vi "A170316-11_Auto.vi"() -> ()   [LabVIEW 2020]
uses:
  Global_Variable/A170316-11.vi
  Global_Variable/Global.vi
  Database/Global1.vi
  <vilib>/addons/database/Connection.llb/DB Tools Open Connec (String).vi
  <vilib>/addons/database/NI_Database_API.lvlib
panel:
  in  "前序OK？_ECU":string
  in  "前序OK？":string
  out "磨合次数":i32
  in  "判定结果":bool[][](array[boolean])=[[TRUE]]
  in  "STEP3":string
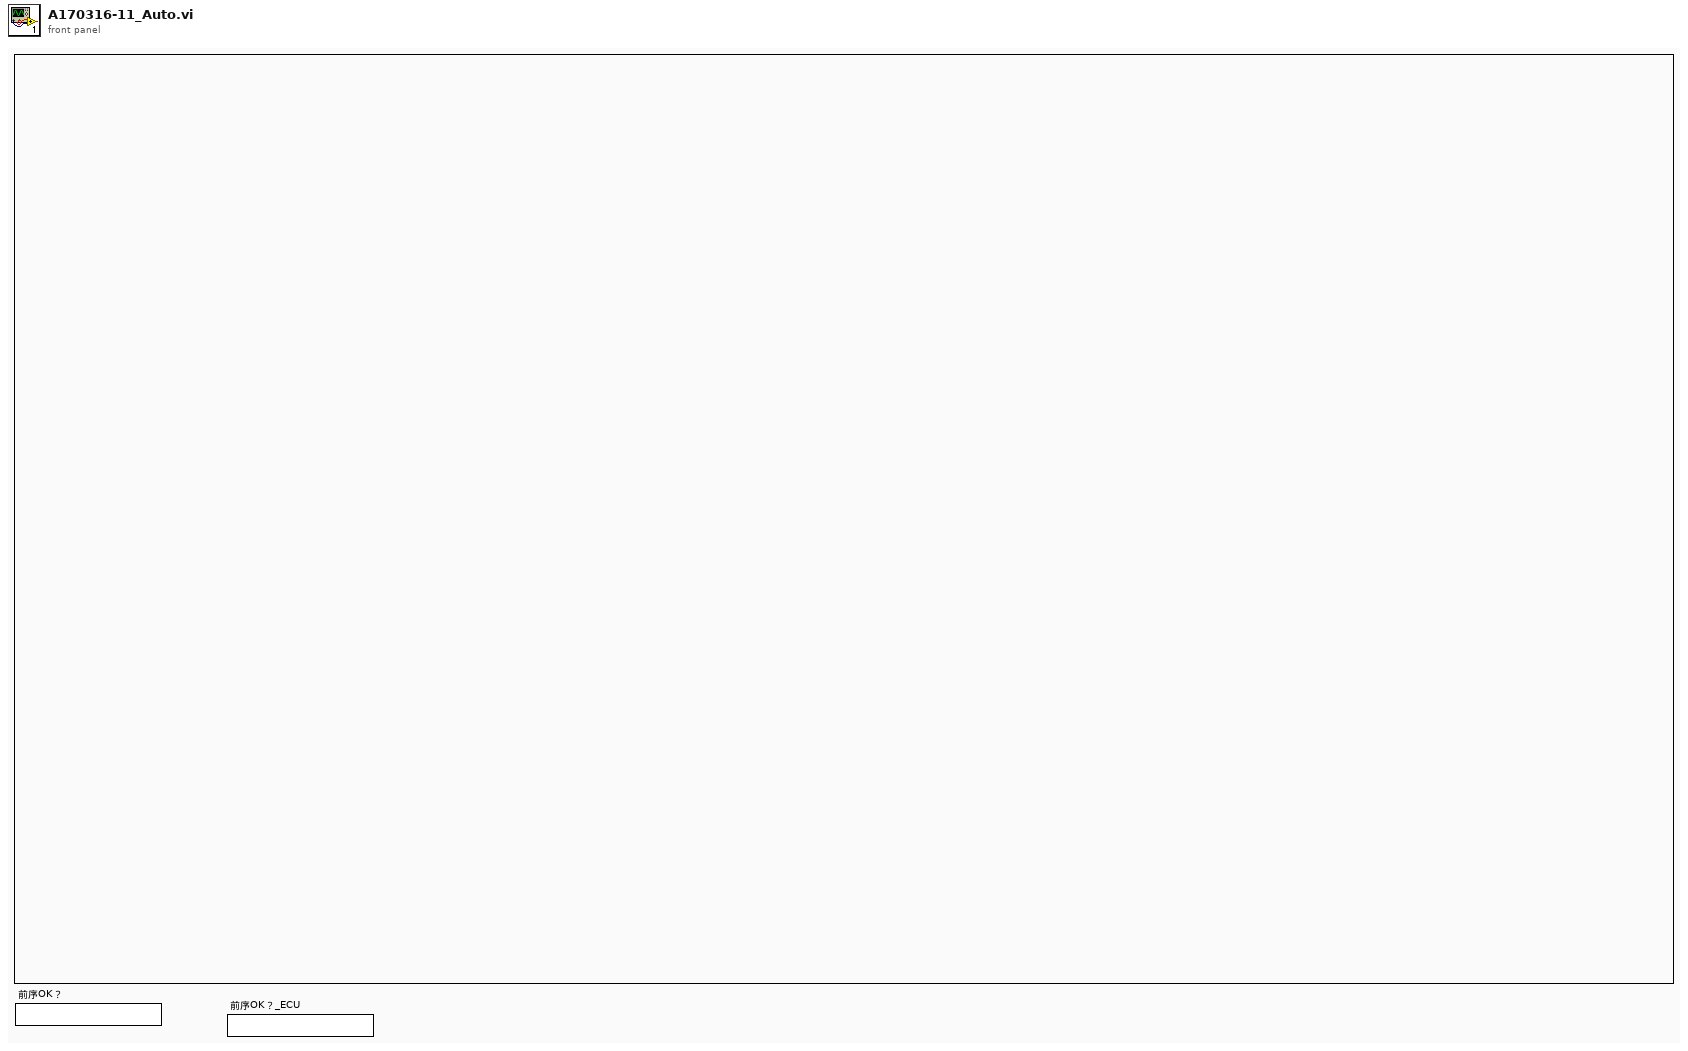
[diagram p1: front panel]
types:
  T1 = cluster{i64, i64, i64, "生产结果":string, "result string":string}
  T2 = cluster{i64, i64, i64, "生产结果":string, "result string":string}[]
  T3 = typedef "NI_Database_API.lvlib/Conn ObjectReference.ctl" = refnum<k1>
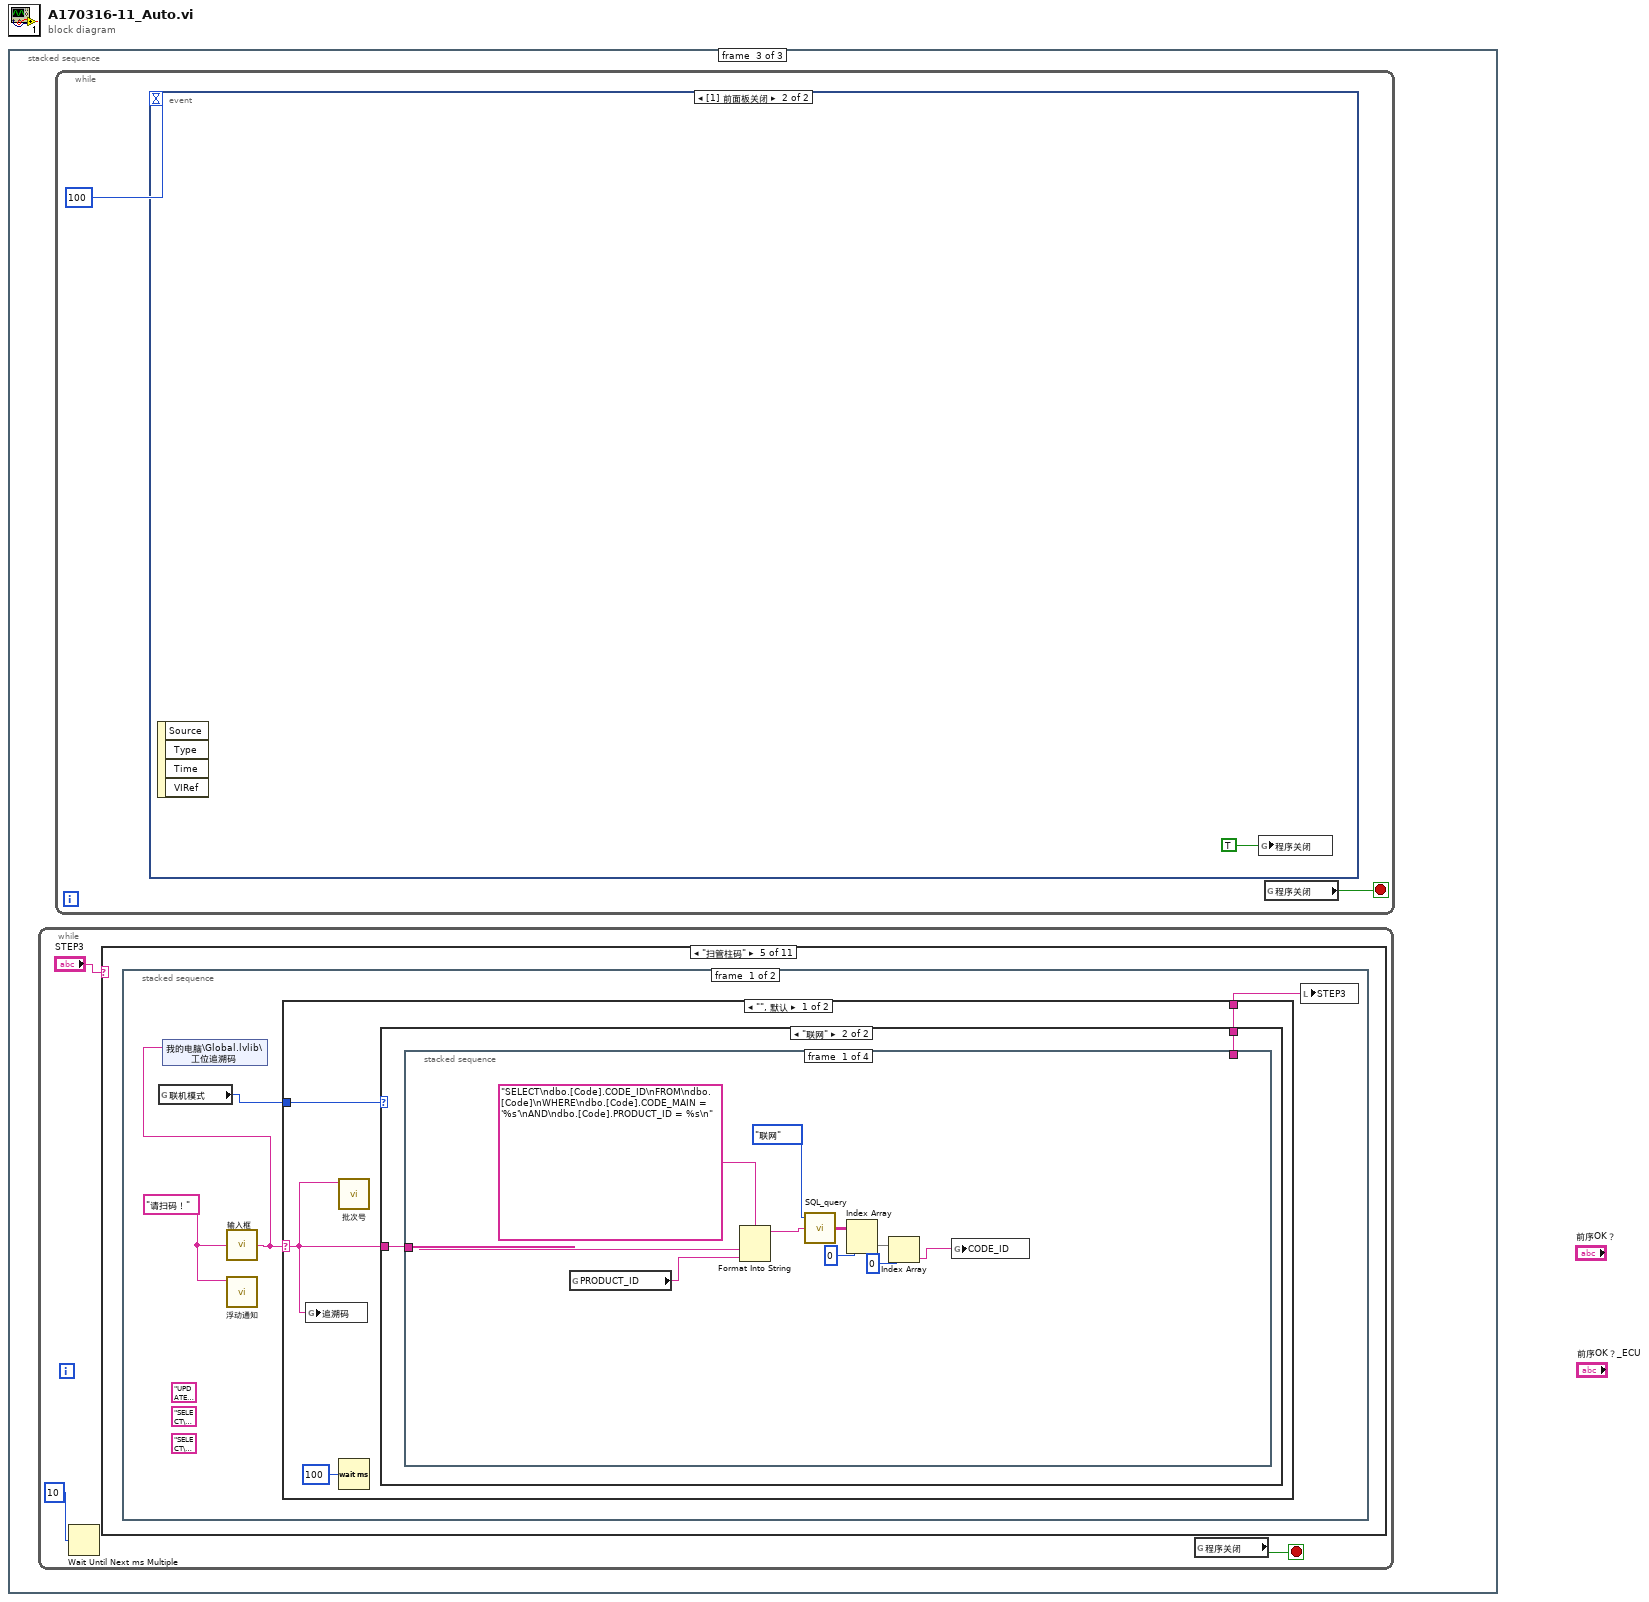
[diagram p0: block diagram]
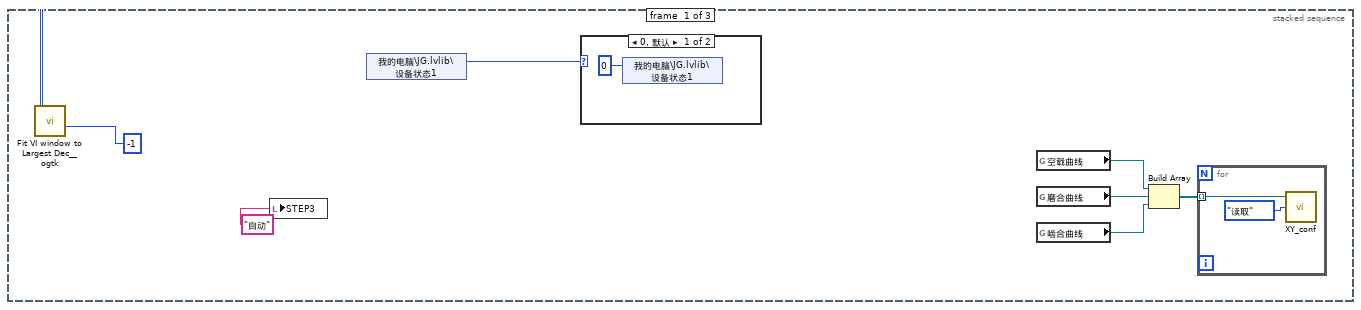
[diagram p2: hidden frame]
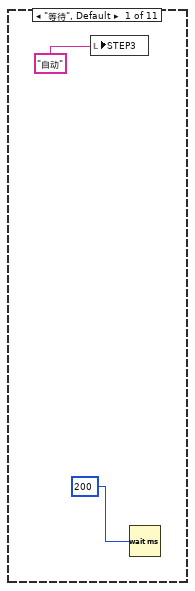
[diagram p5: hidden frame]
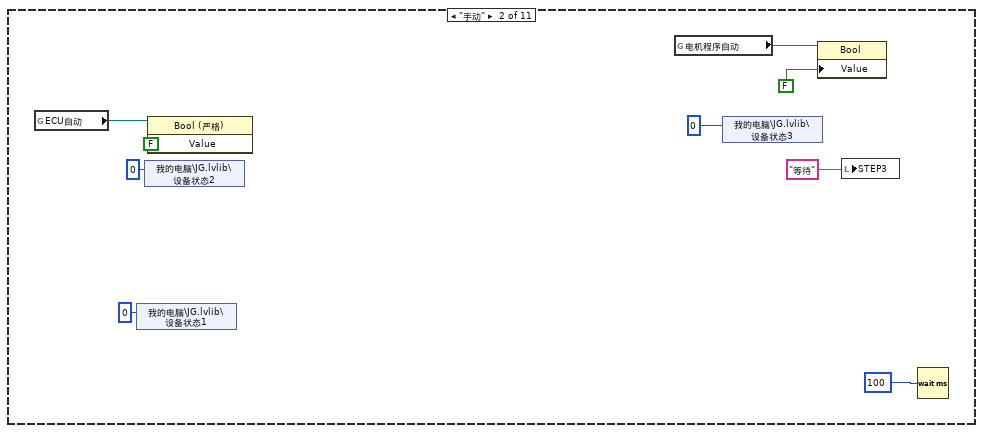
[diagram p6: hidden frame]
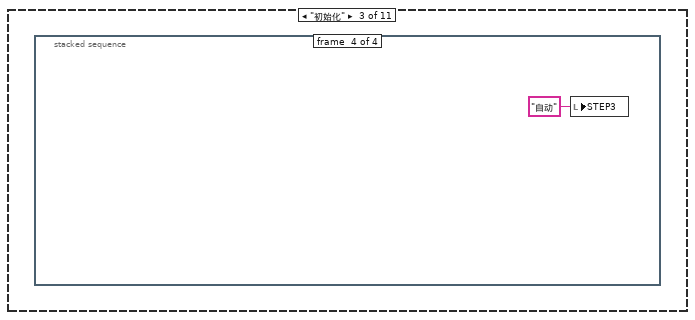
[diagram p7: hidden frame]
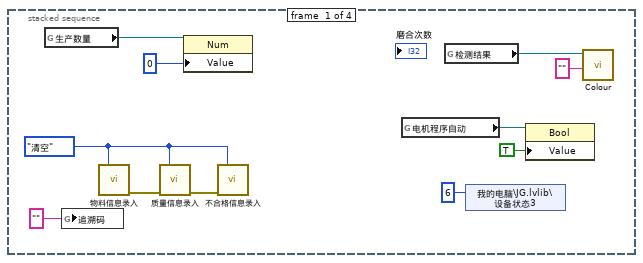
[diagram p8: hidden frame]
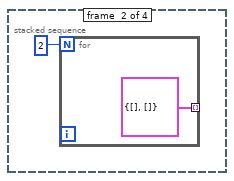
[diagram p9: hidden frame]
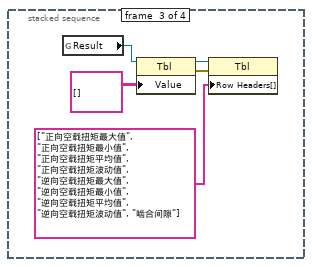
[diagram p10: hidden frame]
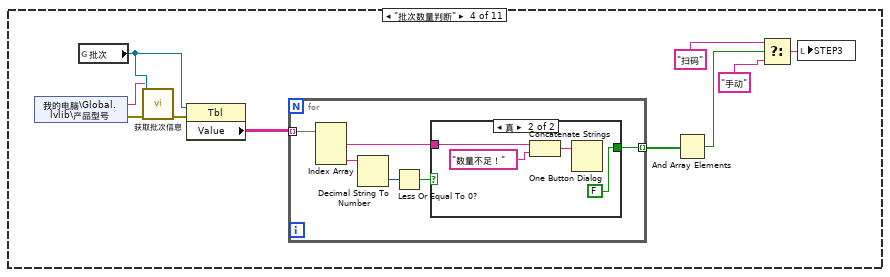
[diagram p11: hidden frame]
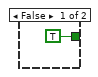
[diagram p12: hidden frame]
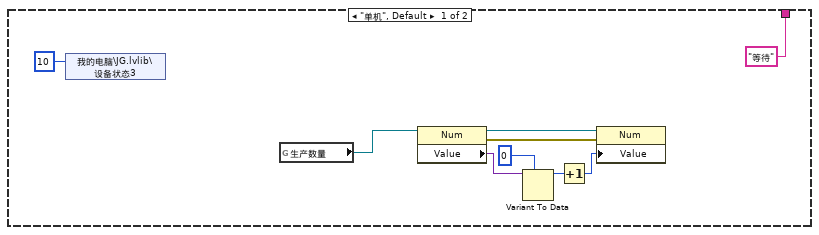
[diagram p13: hidden frame]
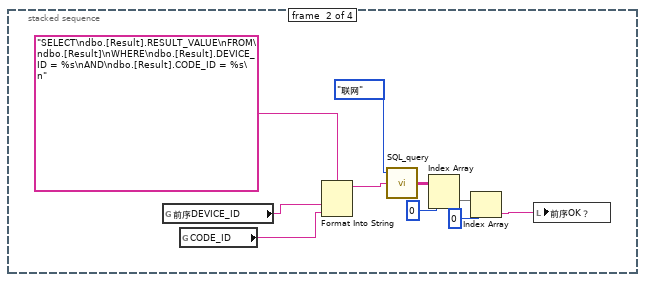
[diagram p14: hidden frame]
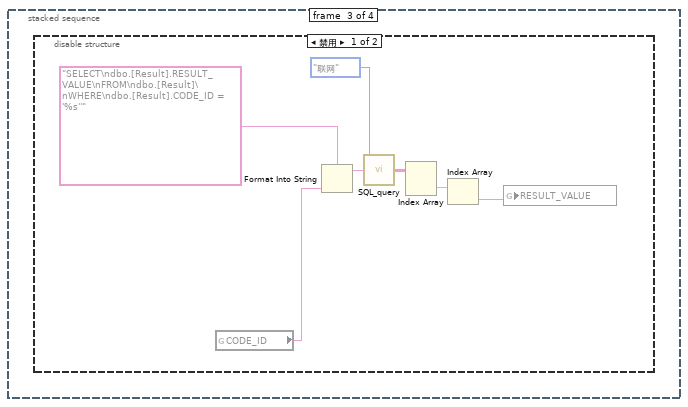
[diagram p15: hidden frame]
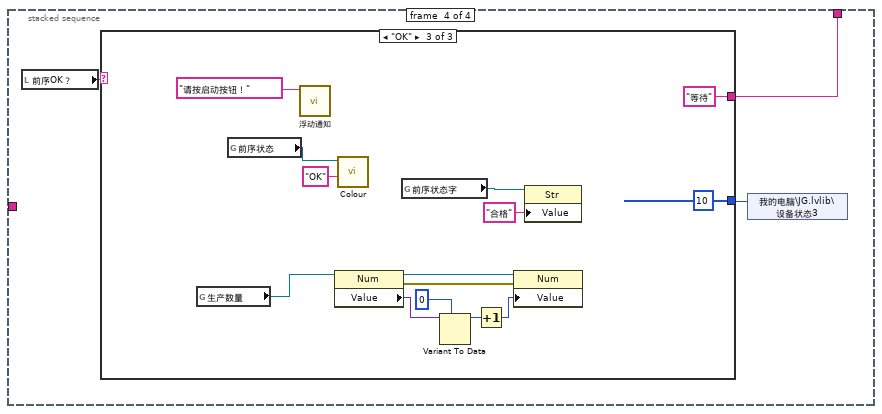
[diagram p17: hidden frame]
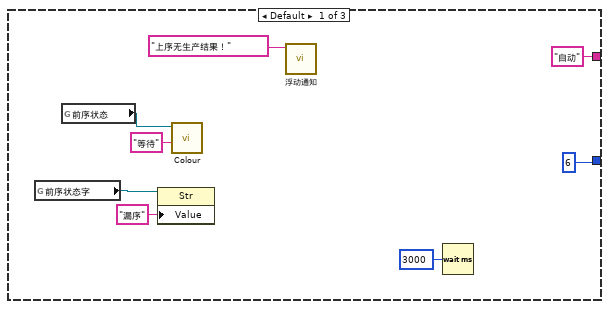
[diagram p18: hidden frame]
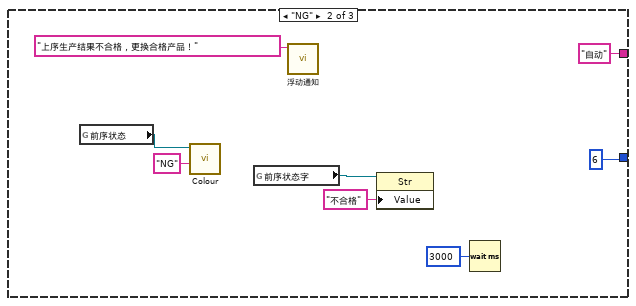
[diagram p19: hidden frame]
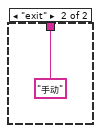
[diagram p20: hidden frame]
diagram:
  n1 = stacked-sequence {
    frame #0 {
      n2 = call <userlib>:"Fit VI window to Largest Dec__ogtk.vi"("border spacing (2 px)"=-1) -> ()  [unwired: 5 in, 2 out]
      n3 = local write "STEP3"("自动" ("STEP")) -> ()
      n4 = shared-variable "我的电脑\\JG.lvlib\\设备状态1"() -> (w5:i16)  [unwired: 1 in, 1 out]
      n5 = case shown="0, 默认" w5 {
        frame 0, Default {
          n6 = shared-variable "我的电脑\\JG.lvlib\\设备状态1"(i16 0 ("设备状态")) -> ()  [unwired: 1 in, 1 out]
        }
        frame 3721..3723 {
        }
      }
      n7 = global read "A170316-11.vi" "空载曲线"() -> (w1:refnum<vi>)
      n8 = global read "A170316-11.vi" "磨合曲线"() -> (w2:refnum<vi>)
      n9 = global read "A170316-11.vi" "啮合曲线"() -> (w3:refnum<vi>)
      n10 = Build Array(w1, w2, w3) -> (w6:refnum<vi>[])
      n11 = for {
        tunnel: w6 -> [w10] mode=indexing
        n12 = call "XY_conf.vi"("方式"=enum16{"写入", "读取"}."读取", "XY图引用"=w10) -> ()  [unwired: 3 in, 1 out]
      }
    }
    frame #1 {
    }
    frame #2 {
      n13 = while {
        stop <- w12 stop-if-true
        n14 = Wait Until Next ms Multiple(millisecond multiple=u32 10 ("毫秒倍数")) -> ()  [unwired: 1 out]
        n15 = case shown="\"扫管柱码\"" "STEP3" {
          frame "等待", Default {
            n16 = local write "STEP3"("自动" ("STEP")) -> ()
            n17 = Wait (ms)(milliseconds to wait=u32 200 ("等待时间（毫秒）")) -> ()  [unwired: 1 out]
          }
          frame "手动" {
            n18 = global read "Global.vi" "ECU自动"() -> (w19:refnum<vi>)
            n19 = shared-variable "我的电脑\\JG.lvlib\\设备状态1"(u16 0 ("设备状态")) -> ()  [unwired: 1 in, 1 out]
            n20 = shared-variable "我的电脑\\JG.lvlib\\设备状态2"(u16 0 ("设备状态")) -> ()  [unwired: 1 in, 1 out]
            n21 = property class="Bool (严格)"(reference=w19, "Value"=FALSE) -> ()  [unwired: 1 in, 2 out]
            n22 = global read "Global.vi" "电机程序自动"() -> (w22:refnum<vi>)
            n23 = shared-variable "我的电脑\\JG.lvlib\\设备状态3"(u16 0 ("设备状态")) -> ()  [unwired: 1 in, 1 out]
            n24 = property class="Bool"(reference=w22, "Value"=FALSE) -> ()  [unwired: 1 in, 2 out]
            n25 = local write "STEP3"("等待" ("STEP")) -> ()
            n26 = Wait (ms)(milliseconds to wait=u32 100 ("等待时间（毫秒）")) -> ()  [unwired: 1 out]
          }
          frame "初始化" {
            n27 = stacked-sequence {
              frame #0 {
                w34 = enum16{"录入", "清空"}."清空" ("功能")
                n28 = global read "Global.vi" "生产数量"() -> (w28:refnum<vi>)
                n29 = global write "Global1.vi" "追溯码"("" ("传感器码")) -> ()
                n30 = call "物料信息录入.vi"("功能"=w34) -> ("错误输出"=w33:errorcluster)  [unwired: 14 in]
                n31 = call "质量信息录入.vi"("功能"=w34, "错误输入（无错误）"=w33) -> ("错误输出"=w35:errorcluster)  [unwired: 13 in]
                n32 = property class="Num"(reference=w28, "Value"=0 ("磨合次数")) -> ()  [unwired: 1 in, 2 out]
                n33 = call "不合格信息录入.vi"("功能"=w34, "错误输入（无错误）"=w35) -> ()  [unwired: 13 in, 1 out]
                n34 = global read "Global.vi" "电机程序自动"() -> (w32:refnum<vi>)
                n35 = global read "Global.vi" "检测结果"() -> (w30:refnum<vi>)
                n36 = shared-variable "我的电脑\\JG.lvlib\\设备状态3"(i16 6 ("设备状态")) -> ()  [unwired: 1 in, 1 out]
                n37 = property class="Bool"(reference=w32, "Value"=TRUE) -> ()  [unwired: 1 in, 2 out]
                n38 = call "Colour.vi"("result"="", "colourRef"=w30) -> ()  [unwired: 9 in, 1 out]
              }
              frame #1 {
                n39 = for {
                  N: 2 -> [_]
                  tunnel: [cluster{dbl[], dbl[]} {[], []}] -> _ mode=indexing
                }
              }
              frame #2 {
                n40 = global read "Global.vi" "Result"() -> (w40:refnum<vi>)
                n41 = property class="Tbl"(reference=w40, "Value"=string[][] []) -> (reference out=w41:refnum<vi>, error out=w42:errorcluster)  [unwired: 1 in]
                n42 = property class="Tbl"(reference=w41, error in=w42, "Row Headers[]"=string[] ["正向空载扭矩最大值", "正向空载扭矩最小值", "正向空载扭矩平均值", "正向空载扭矩波动值", "逆向空载扭矩最大值", "逆向空载扭矩最小值", "逆向空载扭矩平均值", "逆向空载扭矩波动值", "啮合间隙"] ("列首字符串[]")) -> ()  [unwired: 2 out]
              }
              frame #3 {
                n43 = local write "STEP3"("自动" ("STEP")) -> ()
              }
            }
          }
          frame "批次数量判断" {
            n44 = shared-variable "我的电脑\\Global.lvlib\\产品型号"() -> (w49:string, error out=w52:errorcluster)  [unwired: 1 in]
            n45 = global read "Global.vi" "批次"() -> (w50:refnum<vi>)
            n46 = call "获取批次信息.vi"("error in (no error)"=w52, "产品型号"=w49, "Tbl引用句柄"=w50) -> ("error out"=w51:errorcluster)  [unwired: 7 in, 1 out]
            n47 = property class="Tbl"(reference=w50, error in=w51) -> ("Value"=w53:string[][])  [unwired: 2 out]
            n48 = for {
              tunnel: w53 -> [w59] mode=indexing
              tunnel: [w54] -> w48 mode=indexing
              n49 = Index Array(array=w59) -> (element #1=w55:string, element #3=w58:string)  [unwired: 3 in, 1 out]
              n50 = Decimal String To Number(string=w58) -> (number=w57:i32)  [unwired: 2 in, 1 out]
              n51 = Less Or Equal To 0?(x=w57) -> (x <= 0?=w56:bool)
              n52 = case shown="真" w56 {
                tunnel: w55 -> [_ w64]
                tunnel: [TRUE FALSE] -> w54
                frame False {
                }
                frame True {
                  n53 = Concatenate Strings(w64, "数量不足！" ("字符串")) -> (w62:string)
                  n54 = One Button Dialog(message=w62) -> ()  [unwired: 1 in, 1 out]
                }
              }
            }
            n55 = And Array Elements(Boolean array=w48) -> (logical AND=w47:bool)
            n56 = Select(t="扫码" ("STEP"), s=w47, f="手动" ("STEP")) -> (s? t:f=w44:string)
            n57 = local write "STEP3"(w44) -> ()
          }
          frame "扫管柱码" {
            n58 = stacked-sequence {
              frame #0 {
                (unwired) "SELECT\ndbo.[Code].CODE_ID,\ndbo.[Code].CODE_MAIN,\ndbo.[Code].PRODUCT_ID\n\nFROM\ndbo.[Code].CODE_MAIN = 'MACAU3001'" ("格式字符串")
                (unwired) "SELECT\n*\nFROM\ndbo.[Code]\nWHERE\ndbo.[Code].CODE_MAIN = 'MACAU3001'" ("格式字符串")
                (unwired) "UPDATE\ndbo.[Code]\nSET dbo.[Code].CODE_SENSOR = 'henglong'\nWHERE\ndbo.[Code].CODE_MAIN = 'MACAU3001'\n" ("格式字符串")
                w68 = "请扫码！" ("提示信息")
                n59 = global read "Global1.vi" "联机模式"() -> (w66:enum16{"单机", "联网"})
                n60 = call "输入框.vi"("提示信息"=w68) -> ("条形码输出"=w65:string)
                n61 = shared-variable "我的电脑\\Global.lvlib\\工位追溯码"(w65) -> ()  [unwired: 1 in, 1 out]
                n62 = call "浮动通知.vi"("通知内容"=w68) -> ()  [unwired: 11 in]
                n63 = case shown="\"\", 默认" w65 {
                  selector: w65 -> [w69 _]
                  tunnel: [w71 "手动"] -> w67
                  tunnel: w66 -> [w70 _]
                  frame "", Default {
                    n64 = global write "Global1.vi" "追溯码"(w69) -> ()
                    n65 = call "批次号.vi"("批次码"=w69) -> ()  [unwired: 11 in]
                    n66 = Wait (ms)(milliseconds to wait=u32 100 ("等待时间（毫秒）")) -> ()  [unwired: 1 out]
                    n67 = case shown="\"联网\"" w70 {
                      tunnel: w69 -> [_ w83]
                      tunnel: ["等待" ("State(s) in Front (\"\")") w82] -> w71
                      frame "单机", Default {
                        n68 = shared-variable "我的电脑\\JG.lvlib\\设备状态3"(i16 10 ("设备状态控制字")) -> ()  [unwired: 1 in, 1 out]
                        n69 = global read "Global.vi" "生产数量"() -> (w75:refnum<vi>)
                        n70 = property class="Num"(reference=w75) -> (reference out=w73:refnum<vi>, error out=w77:errorcluster, "Value"=w78:variant)  [unwired: 1 in]
                        n71 = Variant To Data(type=u32 0, Variant=w78) -> (data=w79:u32)  [unwired: 1 in, 1 out]
                        n72 = Increment(x=w79) -> (x+1=w80:u32)
                        n73 = property class="Num"(reference=w73, error in=w77, "Value"=w80) -> ()  [unwired: 2 out]
                      }
                      frame "联网" {
                        n74 = stacked-sequence {
                          tunnel: w83 -> [w90 _ _ _]
                          tunnel: [_ _ _ w112] -> w82
                          frame #0 {
                            n75 = global read "Global1.vi" "PRODUCT_ID"() -> (w87:string)
                            n76 = Format Into String(format string="SELECT\ndbo.[Code].CODE_ID\nFROM\ndbo.[Code]\nWHERE\ndbo.[Code].CODE_MAIN = '%s'\nAND\ndbo.[Code].PRODUCT_ID = %s\n" ("格式字符串"), w90, w87) -> (resulting string=w89:string)  [unwired: 2 in, 1 out]
                            n77 = call "SQL_query.vi"("SQL query"=w89, "联机模式"=enum16{"单机", "联网"}."联网") -> ("data"=w93:string[][])  [unwired: 1 in, 2 out]
                            n78 = Index Array(array=w93, index (row)=0 ("索引 (行)")) -> (element=w92:string[])  [unwired: 1 in]
                            n79 = Index Array(array=w92, index=0 ("索引")) -> (element=w84:string)
                            n80 = global write "Global1.vi" "CODE_ID"(w84) -> ()
                          }
                          frame #1 {
                            n81 = global read "Global1.vi" "前序DEVICE_ID"() -> (w95:string)
                            n82 = global read "Global1.vi" "CODE_ID"() -> (w94:string)
                            n83 = Format Into String(format string="SELECT\ndbo.[Result].RESULT_VALUE\nFROM\ndbo.[Result]\nWHERE\ndbo.[Result].DEVICE_ID = %s\nAND\ndbo.[Result].CODE_ID = %s\n" ("格式字符串"), w95, w94) -> (resulting string=w100:string)  [unwired: 2 in, 1 out]
                            n84 = call "SQL_query.vi"("SQL query"=w100, "联机模式"=enum16{"单机", "联网"}."联网") -> ("data"=w103:string[][])  [unwired: 1 in, 2 out]
                            n85 = Index Array(array=w103, index (row)=0 ("索引 (行)")) -> (element=w102:string[])  [unwired: 1 in]
                            n86 = Index Array(array=w102, index=0 ("索引")) -> (element=w96:string)
                            n87 = local write "前序OK？"(w96) -> ()
                          }
                          frame #2 {
                            n88 = disable-structure shown="禁用" {
                              frame Disabled {
                                n89 = global read "Global1.vi" "CODE_ID"() -> (w105:string)
                                n90 = Format Into String(format string="SELECT\ndbo.[Result].RESULT_VALUE\nFROM\ndbo.[Result]\nWHERE\ndbo.[Result].CODE_ID = '%s''" ("格式字符串"), w105) -> (resulting string=w107:string)  [unwired: 2 in, 1 out]
                                n91 = call "SQL_query.vi"("SQL query"=w107, "联机模式"=enum16{"单机", "联网"}."联网") -> ("data"=w110:string[][])  [unwired: 1 in, 2 out]
                                n92 = Index Array(array=w110) -> (element=w108:string[])  [unwired: 2 in]
                                n93 = Index Array(array=w108) -> (element=w109:string)  [unwired: 1 in]
                                n94 = global write "Global1.vi" "RESULT_VALUE"(w109) -> ()
                              }
                              frame Enabled {
                              }
                            }
                          }
                          frame #3 {
                            n95 = local read "前序OK？"() -> (w111:string)
                            n96 = case shown="\"OK\"" w111 {
                              tunnel: [i16 6 ("设备状态控制字") i16 6 ("设备状态控制字") i16 10 ("设备状态控制字")] -> w113
                              tunnel: ["自动" "自动" "等待"] -> w112
                              frame Default {
                                n97 = global read "Global1.vi" "前序状态字"() -> (w115:refnum<vi>)
                                n98 = global read "Global1.vi" "前序状态"() -> (w117:refnum<vi>)
                                n99 = property class="Str"(reference=w115, "Value"="漏序" ("值")) -> ()  [unwired: 1 in, 2 out]
                                n100 = call "Colour.vi"("result"="等待", "colourRef"=w117) -> ()  [unwired: 9 in, 1 out]
                                n101 = call "浮动通知.vi"("通知内容"="上序无生产结果！" ("Status")) -> ()  [unwired: 11 in]
                                n102 = Wait (ms)(milliseconds to wait=u32 3000) -> ()  [unwired: 1 out]
                              }
                              frame "NG" {
                                n103 = global read "Global1.vi" "前序状态"() -> (w125:refnum<vi>)
                                n104 = call "Colour.vi"("result"="NG", "colourRef"=w125) -> ()  [unwired: 9 in, 1 out]
                                n105 = global read "Global1.vi" "前序状态字"() -> (w123:refnum<vi>)
                                n106 = call "浮动通知.vi"("通知内容"="上序生产结果不合格，更换合格产品！" ("Status")) -> ()  [unwired: 11 in]
                                n107 = property class="Str"(reference=w123, "Value"="不合格" ("值")) -> ()  [unwired: 1 in, 2 out]
                                n108 = Wait (ms)(milliseconds to wait=u32 3000) -> ()  [unwired: 1 out]
                              }
                              frame "OK" {
                                n109 = global read "Global.vi" "生产数量"() -> (w141:refnum<vi>)
                                n110 = global read "Global1.vi" "前序状态"() -> (w133:refnum<vi>)
                                n111 = call "浮动通知.vi"("通知内容"="请按启动按钮！" ("Status")) -> ()  [unwired: 11 in]
                                n112 = property class="Num"(reference=w141) -> (reference out=w142:refnum<vi>, error out=w140:errorcluster, "Value"=w139:variant)  [unwired: 1 in]
                                n113 = call "Colour.vi"("result"="OK", "colourRef"=w133) -> ()  [unwired: 9 in, 1 out]
                                n114 = global read "Global1.vi" "前序状态字"() -> (w131:refnum<vi>)
                                n115 = Variant To Data(type=u32 0, Variant=w139) -> (data=w138:u32)  [unwired: 1 in, 1 out]
                                n116 = Increment(x=w138) -> (x+1=w137:u32)
                                n117 = property class="Num"(reference=w142, error in=w140, "Value"=w137) -> ()  [unwired: 2 out]
                                n118 = property class="Str"(reference=w131, "Value"="合格" ("值")) -> ()  [unwired: 1 in, 2 out]
                              }
                            }
                            n119 = shared-variable "我的电脑\\JG.lvlib\\设备状态3"(w113) -> ()  [unwired: 1 in, 1 out]
                          }
                        }
                      }
                    }
                  }
                  frame "exit" {
                  }
                }
                n120 = local write "STEP3"(w67) -> ()
              }
              frame #1 {
                n121 = Wait (ms)(milliseconds to wait=u32 100 ("等待时间（毫秒）")) -> ()  [unwired: 1 out]
              }
            }
          }
          frame "扫电机码" {
            n122 = stacked-sequence {
              frame #0 {
                w146 = "请扫管柱码！" ("提示信息")
                n123 = call "输入框.vi"("提示信息"=w146) -> ("条形码输出"=w147:string)
                n124 = call "浮动通知.vi"("通知内容"=w146) -> ()  [unwired: 11 in]
                n125 = case shown="\"\", 默认" w147 {
                  selector: w147 -> [w149 _]
                  tunnel: [w150 "手动"] -> w148
                  frame "", Default {
                    n126 = global read "Global1.vi" "联机模式"() -> (w151:enum16{"单机", "联网"})
                    n127 = shared-variable "我的电脑\\Global.lvlib\\电机码"(w149) -> ()  [unwired: 1 in, 1 out]
                    n128 = case shown="\"联网\"" w151 {
                      tunnel: w149 -> [_ _]
                      tunnel: ["等待" ("State(s) in Front (\"\")") w155] -> w150
                      frame "单机", Default {
                        n129 = shared-variable "我的电脑\\JG.lvlib\\设备状态3"(i16 35 ("设备状态控制字")) -> ()  [unwired: 1 in, 1 out]
                        n130 = Wait (ms)(milliseconds to wait=u32 100 ("等待时间（毫秒）")) -> ()  [unwired: 1 out]
                      }
                      frame "联网" {
                        n131 = stacked-sequence {
                          tunnel: [_ _ "等待" ("State(s) in Front (\"\")")] -> w155
                          frame #0 {
                          }
                          frame #1 {
                          }
                          frame #2 {
                            n132 = shared-variable "我的电脑\\JG.lvlib\\设备状态3"(i16 35 ("设备状态控制字")) -> ()  [unwired: 1 in, 1 out]
                          }
                        }
                      }
                    }
                  }
                  frame "exit" {
                  }
                }
                n133 = local write "STEP3"(w148) -> ()
              }
              frame #1 {
                n134 = Wait (ms)(milliseconds to wait=u32 100 ("等待时间（毫秒）")) -> ()  [unwired: 1 out]
              }
            }
          }
          frame "录入批次" {
            n135 = shared-variable "我的电脑\\Global.lvlib\\产品型号"() -> (w161:string)  [unwired: 1 in, 1 out]
            n136 = call "更新批次.vi"("型号"=w161) -> ("error out"=w162:errorcluster)  [unwired: 10 in]
            n137 = call "更新易损件.vi"("error in (no error)"=w162) -> ("error out"=w165:errorcluster)  [unwired: 10 in]
            n138 = global read "Global.vi" "批次"() -> (w163:refnum<vi>)
            n139 = property class="Tbl"(reference=w163, error in=w165) -> ("Value"=w164:string[][])  [unwired: 2 out]
            n140 = for {
              tunnel: w164 -> [w168] mode=indexing
              n141 = Index Array(array=w168) -> (element #1=w167:string, element #2=w166:string)  [unwired: 2 in]
              n142 = call "物料信息录入.vi"("物料名称"=w167, "功能"=enum16{"录入", "清空"}."录入", "物料编码"=w166) -> ()  [unwired: 12 in, 1 out]
            }
            n143 = local write "STEP3"("等待" ("STEP")) -> ()
          }
          frame "自动" {
            n144 = shared-variable "我的电脑\\JG.lvlib\\设备状态3"() -> (w170:i16)  [unwired: 1 in, 1 out]
            n145 = case shown="100, 200" w170 {
              frame Default {
              }
              frame -128 {
                n146 = call "浮动通知.vi"("通知内容"="复位中……" ("Status")) -> ()  [unwired: 11 in]
                n147 = global read "Global.vi" "电机程序自动"() -> (w172:refnum<vi>)
                n148 = property class="Bool"(reference=w172, "Value"=FALSE) -> ()  [unwired: 1 in, 2 out]
              }
              frame 5 {
                n149 = call "浮动通知.vi"("通知内容"="复位完成" ("Status")) -> ()  [unwired: 11 in]
              }
              frame 6 {
                n150 = local write "STEP3"("扫管柱码") -> ()
              }
              frame 0 {
              }
              frame 7 {
                n151 = global read "Global.vi" "电机结果显示"() -> (w179:refnum<vi>)
                n152 = shared-variable "我的电脑\\Global.lvlib\\工位追溯码"("" ("传感器码")) -> ()  [unwired: 1 in, 1 out]
                n153 = property class="Str"(reference=w179, "Value"="..." ("结果显示")) -> (reference out=w178:refnum<vi>)  [unwired: 1 in, 1 out]
                n154 = property class="Str"(reference=w178, "Text.TextColor"=u32 16776960) -> ()  [unwired: 1 in, 2 out]
                n155 = local write "STEP3"("扫管柱码" ("STEP3")) -> ()
              }
              frame 8 {
                n156 = call "浮动通知.vi"("通知内容"="程序停止！" ("Status")) -> ()  [unwired: 11 in]
              }
              frame 9 {
                n157 = call "浮动通知.vi"("通知内容"="套花键中" ("Status")) -> ()  [unwired: 11 in]
              }
              frame 11 {
                n158 = call "浮动通知.vi"("通知内容"="主码更新到打标机！" ("Status")) -> ()  [unwired: 11 in]
              }
              frame 12 {
                n159 = call "浮动通知.vi"("通知内容"="已更新到打标机！" ("Status")) -> ()  [unwired: 11 in]
              }
              frame 100, 200 {
                n160 = global read "Global.vi" "电机结果显示"() -> (w189:refnum<vi>)
                n161 = property class="Str"(reference=w189, "Value"=" ..." ("结果显示")) -> (reference out=w188:refnum<vi>)  [unwired: 1 in, 1 out]
                n162 = property class="Str"(reference=w188, "Text.TextColor"=u32 9567230) -> ()  [unwired: 1 in, 2 out]
                n163 = call "浮动通知.vi"("通知内容"="移栽进！" ("Status")) -> ()  [unwired: 11 in]
              }
              frame 300 {
                n164 = call "浮动通知.vi"("通知内容"="防护门下降！" ("Status")) -> ()  [unwired: 11 in]
              }
              frame 400 {
                n165 = call "浮动通知.vi"("通知内容"="启动达标！" ("Status")) -> ()  [unwired: 11 in]
              }
              frame 401 {
                n166 = call "浮动通知.vi"("通知内容"="激光打标中！" ("Status")) -> ()  [unwired: 11 in]
              }
              frame 500 {
                n167 = call "浮动通知.vi"("通知内容"="打标完成！" ("Status")) -> ()  [unwired: 11 in]
              }
              frame 600 {
                n168 = call "浮动通知.vi"("通知内容"="返回！" ("Status")) -> ()  [unwired: 11 in]
              }
              frame 601 {
                n169 = global read "Global1.vi" "联机模式"() -> (w196:enum16{"单机", "联网"})
                n170 = Wait (ms)(milliseconds to wait=u32 500 ("等待时间（毫秒）")) -> ()  [unwired: 1 out]
                n171 = case shown="\"单机\", 默认" w196 {
                  frame "单机", Default {
                    n172 = global read "Global.vi" "检测结果"() -> (w205:refnum<vi>)
                    n173 = call "浮动通知.vi"("通知内容"="产品合格！" ("Status")) -> ()  [unwired: 11 in]
                    n174 = call "Colour.vi"("result"="OK", "colourRef"=w205) -> ()  [unwired: 9 in, 1 out]
                    n175 = global read "Global.vi" "电机结果显示"() -> (w202:refnum<vi>)
                    n176 = property class="Str"(reference=w202, "Value"="OK" ("结果显示")) -> (reference out=w201:refnum<vi>)  [unwired: 1 in, 1 out]
                    n177 = shared-variable "我的电脑\\JG.lvlib\\设备状态3"(i16 6 ("设备状态")) -> ()  [unwired: 1 in, 1 out]
                    n178 = property class="Str"(reference=w201, "Text.TextColor"=u32 65344) -> ()  [unwired: 1 in, 2 out]
                  }
                  frame "联网" {
                    n179 = global read "Global.vi" "检测结果"() -> (w214:refnum<vi>)
                    n180 = global write "Global1.vi" "生产结果"("OK" ("电机工位生产结果")) -> ()
                    n181 = call "浮动通知.vi"("通知内容"="产品合格！" ("Status")) -> ()  [unwired: 11 in]
                    n182 = call "Colour.vi"("result"="OK", "colourRef"=w214) -> ()  [unwired: 9 in, 1 out]
                    n183 = global read "Global.vi" "电机结果显示"() -> (w212:refnum<vi>)
                    n184 = property class="Str"(reference=w212, "Value"="OK" ("结果显示")) -> (reference out=w209:refnum<vi>)  [unwired: 1 in, 1 out]
                    n185 = property class="Str"(reference=w209, "Text.TextColor"=u32 6618880) -> ()  [unwired: 1 in, 2 out]
                    n186 = local write "STEP3"("录入数据库" ("STEP3")) -> ()
                  }
                }
              }
              frame 201 {
                n187 = global read "Global.vi" "检测结果"() -> (w220:refnum<vi>)
                n188 = call "Colour.vi"("result"="NG", "colourRef"=w220) -> ()  [unwired: 9 in, 1 out]
                n189 = call "浮动通知.vi"("通知内容"="产品不合格！" ("Status")) -> ()  [unwired: 11 in]
                n190 = global read "Global.vi" "电机结果显示"() -> (w219:refnum<vi>)
                n191 = property class="Str"(reference=w219, "Value"="NG" ("结果显示")) -> (reference out=w218:refnum<vi>)  [unwired: 1 in, 1 out]
                n192 = property class="Str"(reference=w218, "Text.TextColor"=u32 16711680) -> ()  [unwired: 1 in, 2 out]
              }
              frame 999 {
                n193 = call "浮动通知.vi"("通知内容"="请重新安装固定螺栓！" ("Status")) -> ()  [unwired: 11 in]
                n194 = shared-variable "我的电脑\\JG.lvlib\\设备状态3"(i16 40 ("设备状态")) -> ()  [unwired: 1 in, 1 out]
              }
              frame 1024 {
                n195 = call "浮动通知.vi"("通知内容"="急停！" ("Status")) -> ()  [unwired: 11 in]
                n196 = global read "Global.vi" "电机程序自动"() -> (w225:refnum<vi>)
                n197 = property class="Bool"(reference=w225, "Value"=FALSE) -> ()  [unwired: 1 in, 2 out]
              }
              frame 3721 {
                n198 = local write "STEP3"("不合格锁定" ("STEP")) -> ()
                n199 = call "浮动通知.vi"("通知内容"="产品不合格程序锁定！" ("Status")) -> ()  [unwired: 11 in]
              }
              frame 3722 {
                n200 = global read "Global.vi" "电机程序自动"() -> (w230:refnum<vi>)
                n201 = call "浮动通知.vi"("通知内容"="授权成功，请复位！" ("Status")) -> ()  [unwired: 11 in]
                n202 = property class="Bool"(reference=w230, "Value"=FALSE) -> ()  [unwired: 1 in, 2 out]
              }
              frame 3723 {
                n203 = call "浮动通知.vi"("通知内容"="请取出不合格产品并摆放至不合格品区！" ("Status")) -> ()  [unwired: 11 in]
              }
            }
          }
          frame "录入数据库" {
            n204 = stacked-sequence {
              frame #0 {
                n205 = Get Date/Time String(date format (0)=enum16{"short", "long", "abbreviated"}."short" ("日期格式(0)"), want seconds? (F)=FALSE ("需要秒？(F)")) -> (date string=w242:string, time string=w243:string)  [unwired: 1 in]
                n206 = global read "Global1.vi" "DEVICE_ID"() -> (w246:string)
                n207 = global read "Global1.vi" "USER_ID"() -> (w244:string)
                n208 = global read "Global1.vi" "CODE_ID"() -> (w245:string)
                n209 = global read "Global1.vi" "生产结果"() -> (w237:string)
                n210 = Concatenate Strings(w242, " " ("字符串"), w243) -> (w238:string)
                n211 = Decimal String To Number(string=w246, default (0L)=i64 0 ("默认(0 I32)")) -> (number=w235:i64)  [unwired: 1 in, 1 out]
                n212 = Decimal String To Number(string=w244, default (0L)=i64 0 ("默认(0 I32)")) -> (number=w234:i64)  [unwired: 1 in, 1 out]
                n213 = Decimal String To Number(string=w245, default (0L)=i64 0 ("默认(0 I32)")) -> (number=w233:i64)  [unwired: 1 in, 1 out]
                n214 = global read "Global1.vi" "联机模式"() -> (w253:enum16{"单机", "联网"})
                n215 = Search and Replace String(replace all?=TRUE ("替换全部？(F)"), input string=w238, search string="/" ("替换字符串(\"\")"), replace string="-" ("替换字符串(\"\")")) -> (result string=w236:string)  [unwired: 4 in, 3 out]
                n216 = Bundle(w235, w234, w233, "生产结果"=w237, "result string"=w236) -> (w259:T1)  [unwired: 1 in]
                n217 = call "GetSQLstring.vi"("联机模式"=w253) -> ("错误输出"=w256:errorcluster, "连接字符串"=w255:string)  [unwired: 9 in]
                n218 = Build Array(w259) -> (w260:T2)
                n219 = call-poly <vilib>:"DB Tools Open Connection.vi"("error in (no error)"=w256, "connection information"=w255) -> ("error out"=w254:errorcluster, "connection reference"=w257:T3)  [unwired: 6 in]
                n220 = for {
                  tunnel: w260 -> [w265] mode=indexing
                  tunnel: w257 -> [w263]
                  shift-right: [w261] -> w258
                  shift-left: w254 -> [w268]
                  w264 = string[] ["DEVICE_ID", "USER_ID", "CODE_ID", "RESULT_VALUE", "RESULT_TIME"] ("columns")
                  w266 = "Result" ("table")
                  n221 = call <vilib>:"DB Tools Insert Data.vi"("data"=w265, "error in (no error)"=w268, "columns"=w264, "table"=w266, "connection reference"=w263) -> ("error out"=w267:errorcluster, "connection reference out"=w262:T3)  [unwired: 5 in]
                  n222 = case shown="错误" w267 {
                    selector: w267 -> [w269 w290]
                    tunnel: w264 -> [_ w287]
                    tunnel: w262 -> [w270 w279]
                    tunnel: w266 -> [_ w291]
                    tunnel: w265 -> [_ w283]
                    tunnel: [w270 w278] -> _
                    tunnel: [w269 w277] -> w261
                    frame No Error {
                    }
                    frame Error {
                      n223 = Array Subset(array=w287, index=3 ("长度"), length=2 ("长度")) -> (w288:string[])
                      n224 = Unbundle(w283) -> (w272:i64, w275:i64, "生产结果"=w282:string, "result string"=w281:string)  [unwired: 1 out]
                      n225 = Number To Decimal String(number=w275) -> (decimal integer string=w276:string)  [unwired: 1 in]
                      n226 = Number To Decimal String(number=w272) -> (decimal integer string=w271:string)  [unwired: 1 in]
                      n227 = Concatenate Strings("WHERE CODE_ID =" ("condition"), w276, "AND DEVICE_ID = ", w271) -> (w284:string)
                      n228 = Bundle("生产结果"=w282, "result string"=w281) -> (w280:cluster{"生产结果":string, "result string":string})  [unwired: 1 in]
                      n229 = call <vilib>:"Clear Errors.vi"("error in (no error)"=w290) -> ("error out"=w289:errorcluster)  [unwired: 5 in, 1 out]
                      n230 = call <vilib>:"DB Tools Update Data.vi"("condition"=w284, "data"=w280, "error in (no error)"=w289, "columns"=w288, "table"=w291, "connection reference"=w279) -> ("error out"=w277:errorcluster, "connection reference out"=w278:T3)  [unwired: 4 in]
                    }
                  }
                }
                n231 = call <vilib>:"Simple Error Handler.vi"("error in (no error)"=w258) -> ()  [unwired: 4 in, 5 out]
              }
              frame #1 {
              }
              frame #2 {
              }
              frame #3 {
                n232 = call "浮动通知.vi"("通知内容"="数据录入成功！" ("Status")) -> ()  [unwired: 11 in]
                n233 = shared-variable "我的电脑\\JG.lvlib\\设备状态3"(i16 6 ("设备状态")) -> ()  [unwired: 1 in, 1 out]
                n234 = local write "STEP3"("自动" ("STEP")) -> ()
                n235 = Wait (ms)(milliseconds to wait=u32 1000 ("等待时间（毫秒）")) -> ()  [unwired: 1 out]
              }
            }
          }
          frame "不合格锁定" {
            n236 = call "临时授权.vi"() -> ("授权成功"=w297:bool)  [unwired: 11 in]
            n237 = case shown="真" w297 {
              frame False {
              }
              frame True {
                n238 = local write "STEP3"("报表" ("STEP")) -> ()
                n239 = shared-variable "我的电脑\\JG.lvlib\\设备状态1"(i16 3722 ("设备状态")) -> ()  [unwired: 1 in, 1 out]
              }
            }
            n240 = Wait (ms)(milliseconds to wait=u32 100 ("等待时间（毫秒）")) -> ()  [unwired: 1 out]
          }
          frame "报表" {
            n241 = call "浮动通知.vi"("通知内容"="报表生成中" ("Status")) -> ()  [unwired: 11 in]
            n242 = shared-variable "我的电脑\\Global.lvlib\\工位追溯码"() -> (w309:string)  [unwired: 1 in, 1 out]
            n243 = Index Array(array="判定结果", index (col)=1 ("禁用的索引 (列)")) -> (element=w304:bool[])  [unwired: 1 in]
            n244 = And Array Elements(Boolean array=w304) -> (logical AND=w301:bool)
            n245 = shared-variable "我的电脑\\Global.lvlib\\联机模式"() -> (w306:i16)  [unwired: 1 in, 1 out]
            n246 = case shown="真" w301 {
              frame False {
              }
              frame True {
                n247 = global read "Global.vi" "生产数量"() -> (w318:refnum<vi>)
                n248 = property class="Num"(reference=w318) -> (reference out=w317:refnum<vi>, error out=w316:errorcluster, "Value"=w315:variant)  [unwired: 1 in]
                n249 = Variant To Data(type=u32 0, Variant=w315) -> (data=w314:u32)  [unwired: 1 in, 1 out]
                n250 = Increment(x=w314) -> (x+1=w313:u32)
                n251 = property class="Num"(reference=w317, error in=w316, "Value"=w313) -> ()  [unwired: 2 out]
              }
            }
            n252 = call "Report_A170316-11.vi"("文件重命名"=TRUE, "文件名称"=w309, "布尔数组"="判定结果") -> ("error out"=w307:errorcluster)  [unwired: 8 in]
            n253 = case shown="0, 默认" w306 {
              tunnel: w307 -> [_ w319]
              frame 0, Default {
              }
              frame 1 {
                n254 = call "上传数据库.vi"("错误输入"=w319) -> ()  [unwired: 10 in, 1 out]
              }
            }
            n255 = shared-variable "我的电脑\\JG.lvlib\\设备状态1"() -> (w300:i16)  [unwired: 1 in, 1 out]
            n256 = case shown="3721..3723" w300 {
              frame Default {
                n257 = local write "STEP3"("初始化" ("STEP")) -> ()
              }
              frame 3721..3723 {
                n258 = local write "STEP3"("等待" ("STEP")) -> ()
              }
            }
          }
        }
        n259 = global read "Global.vi" "程序关闭"() -> (w12:bool)
      }
      n260 = while {
        stop <- w320 stop-if-true
        n261 = event shown="[1] 前面板关闭" {
          selector: _ -> [_ _]
          dyn-events: _ -> [_ _]
          timeout: 100 -> [_ _]
          event Timeout {
            n262 = event-data() -> ()  [unwired: 1 in, 3 out]
            n263 = stacked-sequence {
              frame #0 {
                n264 = shared-variable "我的电脑\\JG.lvlib\\错误代码"() -> (w322:u16)  [unwired: 1 in, 1 out]
                n265 = feedback #1() -> (w332:u16)  [unwired: 1 in]
                n266 = feedback-in #1(w322) -> ()
                n267 = Greater Or Equal?(x=w322, y=i16 5000) -> (x >= y?=w330:bool)
                n268 = Less?(x=w322, y=i16 5200) -> (x < y?=w331:bool)
                n269 = Equal?(x=w322, y=w332) -> (x = y?=w329:bool)
                n270 = global read "Global.vi" "报警图标"() -> (w324:refnum<vi>)
                n271 = And(x=w330, y=w331) -> (x .and. y?=w323:bool)
                n272 = property class="Bool"(reference=w324, "Value"=w323) -> ()  [unwired: 1 in, 2 out]
                n273 = Bundle By Name(cluster=errorcluster {"status"=FALSE, "code"=0, "source"=""} ("错误常量"), "status"=w323, "code"=w322) -> (w328:errorcluster)
                n274 = case shown="真" w329 {
                  tunnel: w328 -> [w337 _]
                  frame False {
                    n275 = call "报警处理.vi"("错误常量"=w337) -> ()  [unwired: 9 in, 2 out]
                  }
                  frame True {
                  }
                }
                n276 = case shown="0" w322 {
                  frame 0 {
                    n277 = global read "Global.vi" "报警图标"() -> (w333:refnum<vi>)
                    n278 = property class="Bool"(reference=w333, "Visible"=FALSE ("可见")) -> ()  [unwired: 1 in, 2 out]
                  }
                  frame 1, Default {
                    n279 = global read "Global.vi" "报警图标"() -> (w336:refnum<vi>)
                    n280 = property class="Bool"(reference=w336, "Visible"=TRUE ("可见")) -> ()  [unwired: 1 in, 2 out]
                  }
                }
              }
              frame #1 {
                n281 = disable-structure shown="启用" {
                  frame Disabled {
                    n282 = global read "Global.vi" "ECU自动"() -> (w338:refnum<vi>)
                    n283 = property class="Bool (严格)"(reference=w338) -> ("Value"=w339:bool)  [unwired: 1 in, 2 out]
                    n284 = Variant To Data(type=FALSE, Variant=w339) -> (data=w341:bool)  [unwired: 1 in, 1 out]
                    n285 = case shown="真" w341 {
                      selector: w341 -> [w343 _]
                      frame False {
                        n286 = call <userlib>:"Boolean Trigger__ogtk.vi"("Boolean Input"=w343) -> ("Rising Edge"=w342:bool)  [unwired: 1 in, 1 out]
                        n287 = case shown="假" w342 {
                          frame False {
                          }
                          frame True {
                            n288 = local write "STEP3"("手动" ("STEP")) -> ()
                          }
                        }
                      }
                      frame True {
                        n289 = shared-variable "我的电脑\\JG.lvlib\\设备状态2"() -> (w345:i16)  [unwired: 1 in, 1 out]
                        n290 = case shown="5" w345 {
                          frame 0, Default {
                            n291 = global read "Global.vi" "ECU自动"() -> (w347:refnum<vi>)
                            n292 = property class="Bool (严格)"(reference=w347, "Value"=FALSE) -> ()  [unwired: 1 in, 2 out]
                          }
                          frame 5 {
                            w348 = "初始化" ("STEP")
                            n293 = local write item#-1(w348) -> ()
                            n294 = local write item#-1(w348) -> ()
                          }
                        }
                      }
                    }
                  }
                  frame Enabled {
                  }
                }
                n295 = disable-structure shown="启用" {
                  frame Disabled {
                    n296 = shared-variable "我的电脑\\JG.lvlib\\设备状态3"() -> (w351:i16)  [unwired: 1 in, 1 out]
                    n297 = global read "Global.vi" "电机程序自动"() -> (w350:refnum<vi>)
                    n298 = property class="Bool"(reference=w350) -> ("Value"=w349:variant)  [unwired: 1 in, 2 out]
                    n299 = Variant To Data(type=FALSE, Variant=w349) -> (data=w352:bool)  [unwired: 1 in, 1 out]
                    n300 = case shown="假" w352 {
                      selector: w352 -> [w355 _]
                      tunnel: w351 -> [_ w357]
                      frame False {
                        n301 = call <userlib>:"Boolean Trigger__ogtk.vi"("Boolean Input"=w355) -> ("Rising Edge"=w354:bool)  [unwired: 1 in, 1 out]
                        n302 = case shown="真" w354 {
                          frame False {
                          }
                          frame True {
                            n303 = local write "STEP3"("手动" ("STEP")) -> ()
                          }
                        }
                      }
                      frame True {
                        n304 = case shown="5" w357 {
                          frame 0, Default {
                            n305 = global read "Global.vi" "电机程序自动"() -> (w359:refnum<vi>)
                            n306 = property class="Bool"(reference=w359, "Value"=FALSE) -> ()  [unwired: 1 in, 2 out]
                            n307 = call "浮动通知.vi"("通知内容"="请复位电机装配工位！") -> ()  [unwired: 11 in]
                          }
                          frame 5 {
                            n308 = local write "STEP3"("初始化" ("STEP")) -> ()
                          }
                        }
                      }
                    }
                  }
                  frame Enabled {
                  }
                }
              }
              frame #2 {
              }
            }
          }
          event Panel Close {
            n309 = event-data() -> ()  [unwired: 1 in, 4 out]
            n310 = global write "Global.vi" "程序关闭"(TRUE ("程序关闭")) -> ()
          }
        }
        n311 = global read "Global.vi" "程序关闭"() -> (w320:bool)
      }
    }
  }
